vi "Test shm get Sample scalars LV.vi"(8 "error in (no error)":errorcluster, 11 "scalars_Ctl":T1) -> (0 "error out":errorcluster, 2 "function return":i32, 3 "scalars_Ctl out":T1)   [LabVIEW 2018, in "SALLV_Test.lvlib"]
doc: "int Test_shm_getSample_scalarsLV(Test_scalarsLV *scalars_Ctl );"
uses:
  SALLV_Test.lvlib
  SALLV_Test.so
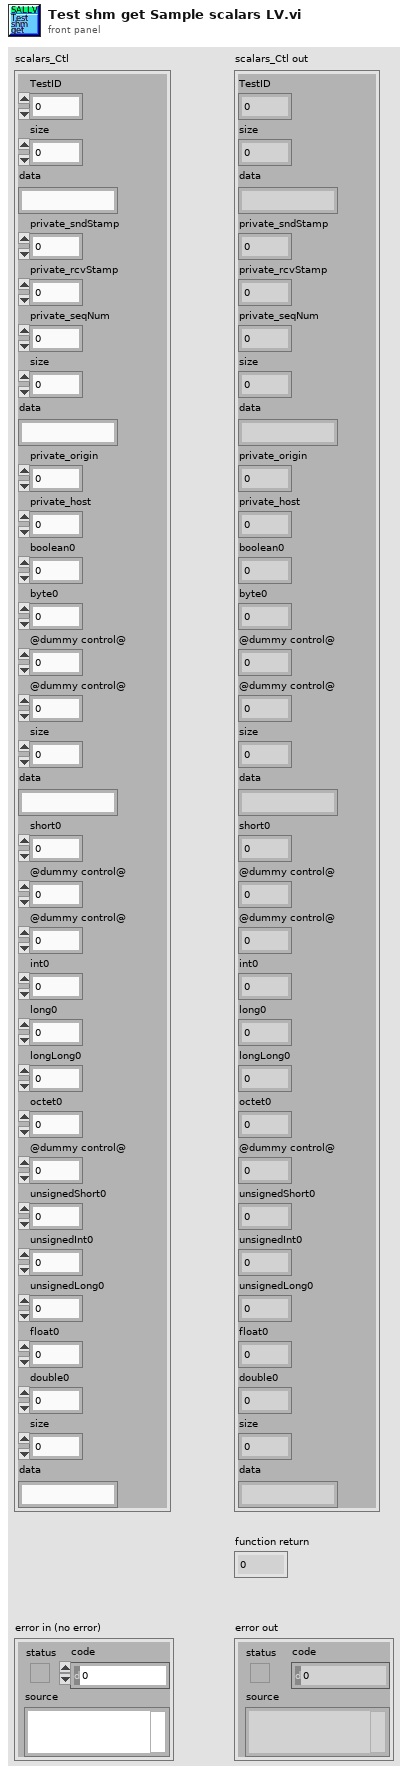
[diagram p1: front panel]
types:
  T1 = cluster{"TestID":i32, "size":i32, "data":string, "private_sndStamp":dbl, "private_rcvStamp":dbl, "private_seqNum":i32, "size":i32, "data":string, "private_origin":i32, "private_host":i32, "boolean0":u8, "byte0":u8, "@dummy control@":i8, "@dummy control@":i8, "size":i32, "data":string, "short0":i16, "@dummy control@":i8, "@dummy control@":i8, "int0":i32, "long0":i32, "longLong0":i32, "octet0":u8, "@dummy control@":i8, "unsignedShort0":u16, "unsignedInt0":u32, "unsignedLong0":u32, "float0":sgl, "double0":dbl, "size":i32, "data":string}
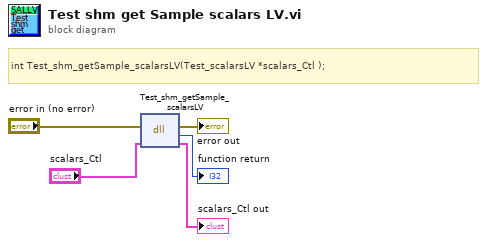
[diagram p0: block diagram]
diagram:
  # "int Test_shm_getSample_scalarsLV(Test_scalarsLV *scalars_Ctl );"
  n1 = dll-call lib="home/ttsai/Documents/salTestLabViewApi/SALLV_Test/SALLV_Test.*" fn="Test_shm_getSample_scalarsLV"(error in="error in (no error)", "scalars_Ctl"="scalars_Ctl") -> (error out=→"error out":errorcluster, →"function return":i32, "scalars_Ctl"=→"scalars_Ctl out":T1)  [unwired: 2 in, 1 out]
